vi "_PC_Pub_XYPlot_Append.vi"(8 "error in (no error)":errorcluster, 10 "spectraData":waveform(sgl)[](array[waveform])) -> (0 "error out":errorcluster, 1 "size(s)":i32, 2 "Spectrum out":cluster{"X":dbl[], "Y":sgl[]})   [LabVIEW 2018]
uses:
  Class/Sig2MS/Sig2MS.lvclass
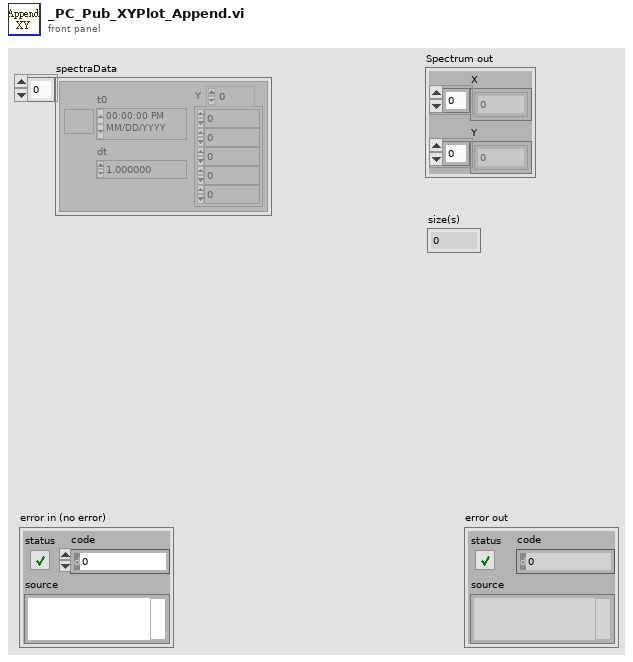
[diagram p1: front panel]
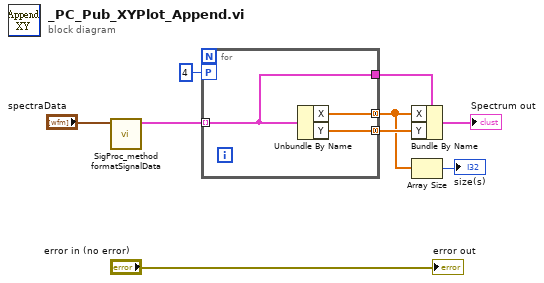
[diagram p0: block diagram]
diagram:
  n1 = call "SigProc_method formatSignalData.vi"("spectraSignal"="spectraData") -> ("spectraData"=w1:cluster{"X":dbl[], "Y":sgl[]}[])  [unwired: 8 in, 2 out]
  n2 = for {
    tunnel: w1 -> [w10] mode=indexing
    tunnel: [w12] -> w6 mode=concatenating
    tunnel: [w11] -> w8 mode=concatenating
    tunnel: [w10] -> w9
    workers-P: 4 -> [_]
    n3 = Unbundle By Name(w10) -> ("X"=w12:dbl[], "Y"=w11:sgl[])
  }
  n4 = Bundle By Name(cluster=w9, "X"=w6, "Y"=w8) -> (→"Spectrum out":cluster{"X":dbl[], "Y":sgl[]})
  n5 = Array Size(array=w6) -> (size(s)=→"size(s)":i32)
  "error out" <- "error in (no error)"
